vi "logging_start.vi"(8 "error in":errorcluster caption="error in (no error)", 11 "VISA resource name":refnum<visa-resource-name>) -> (0 "error out":errorcluster, 3 "VISA resource name out":refnum<visa-resource-name>)   [LabVIEW 2022 SP3, in "hmp4000_rsidr_core.lvlib"]
uses:
  hmp4000_rsidr_core.lvlib
  _type_Logging_Parameter.ctl
  type_Error_Codes.ctl
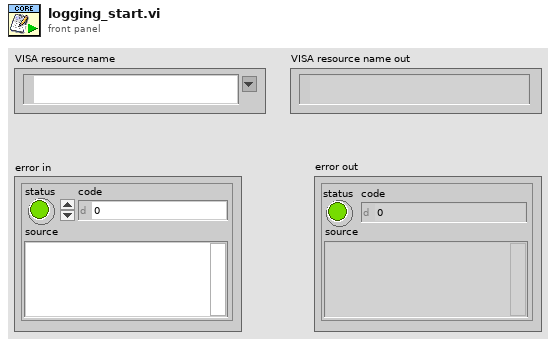
[diagram p1: front panel]
types:
  T1 = typedef "hmp4000_rsidr_core.lvlib/_type_Logging_Parameter.ctl" = enum16{"Type (String)", "SessionAlias(String)", "FormatString (String)", "UDPconectionID (I32)", "UDPlocalPort (I32)", "UDPremotePort (I32)", "UDPremoteHost (String)", "FILEmode (I32)", "FILEpath (String)", "FILEopenID (I32)", "DataMaxLogLen (I32)"}
  T2 = enum16{"open", "replace", "create", "open or create", "replace or create", "replace or create with confirmation"}
  T3 = typedef "hmp4000_rsidr_core.lvlib/type_Error_Codes.ctl" = enum16{"No_error", "VISA_err_ResourceNotFound", "VISA_err_Timeout", "VISA_warn_MoreDataAvailable", "RS_err_MissingCallback", "RS_err_InvalidAttribute", "RS_err_InvalidValue", "RS_err_UnknownResource", "RS_err_AlreadyInitialized", "RS_err_InstrumentStatus", "RS_err_BadRepCapName", "RS_err_TypesMismatch", "RS_err_ValueNotSupported", "RS_err_InvalidRngTable", "RS_err_IDqueryFail", "RS_err_UnexpResponse", "VISA_warn_ConfigNotLoaded", "RS_err_AttributeNotReadable", "RS_err_AttributeNotWritable", "RS_err_InstrumentType", "RS_err_InstrumentOption", "VISA_err_InvalidSize", "RS_err_ReliabilityIndicator", "VISA_warn_UnknownStatus", "VISA_warn_TermCharRead", "VISA_err_IO_error", "RS_err_FunctionNotSupported", "VISA_warn_QueueEmpty"}
  T4 = typedef "hmp4000_rsidr_core.lvlib/type_Session_Data.ctl" = cluster{"IDN string":string, "Instrument FW":string, "Instr type":string, "Instr type for err. msg.":string, "Installed Options":string[], "Ignore Error Messages":string, "Logging params":variant, "OPC Timeout":i32, "VISA Timeout":i32, "STB Poll VISA Timeout":i32, "Additional Flags":i32, "Wait Before Read":i32, "Wait Before Write":i32, "Option String Flags":i32, "IO Segment Size":i64, "VISA Access Mode":T5, "Interface Type":T6, "OPC Wait Mode":T7, "Bin Float Number  Format":T8, "Bin Integer Number Format":T9, "Simulate":bool, "VXIcapable":bool, "Duplicate Session":bool, "Add LF to Write":bool, "Logging":bool, "Fast Sweep":bool, "Query Instrument Status":bool, "Check Range":bool, "Check Options":bool}
  T5 = typedef "hmp4000_rsidr_core.lvlib/type_VisaAccessMode.ctl" = u16
  T6 = typedef "hmp4000_rsidr_core.lvlib/type_InterfaceType.ctl" = enum16{"Unknown", "GPIB", "VXI", "GPIB_VXI", "ASRL", "PXI", "TCPIP", "USB", "SOCKET"}
  T7 = typedef "hmp4000_rsidr_core.lvlib/type_OPC_Wait_Mode.ctl" = enum16{"STBpolling", "STBpollingSlow", "STBpollingSuperSlow", "ServiceRequest", "OPCquery"}
  T8 = typedef "hmp4000_rsidr_core.lvlib/type_Binary_Float_Number_Format.ctl" = enum16{"Float_4_Bytes_Swapped", "Float_4_Bytes", "Double_8_Bytes_Swapped", "Double_8_Bytes"}
  T9 = typedef "hmp4000_rsidr_core.lvlib/type_Binary_Integer_Number_Format.ctl" = enum16{"Int32_4_Bytes_Swapped", "Int32_4 Bytes", "Int16_2_Bytes_Swapped", "Int16_2_Bytes"}
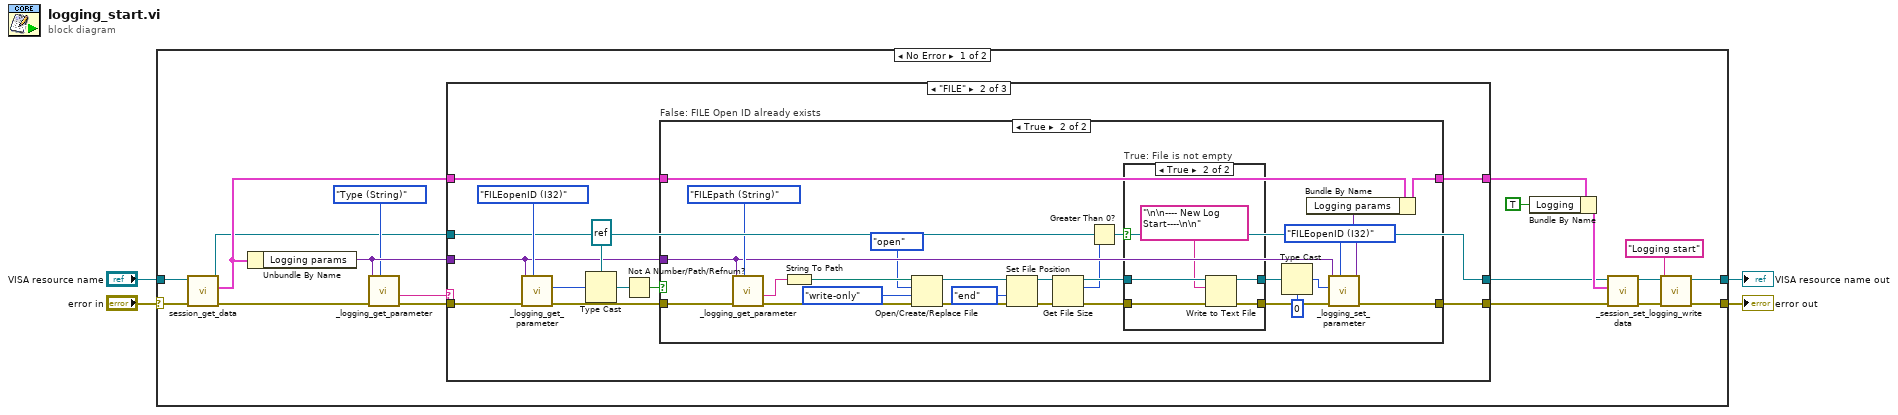
[diagram p0: block diagram]
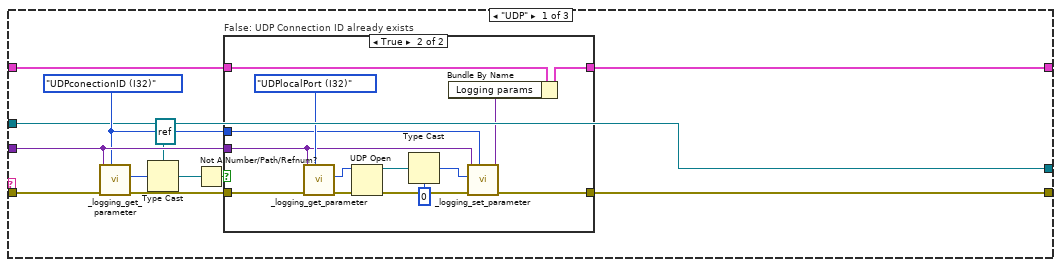
[diagram p2: hidden frame]
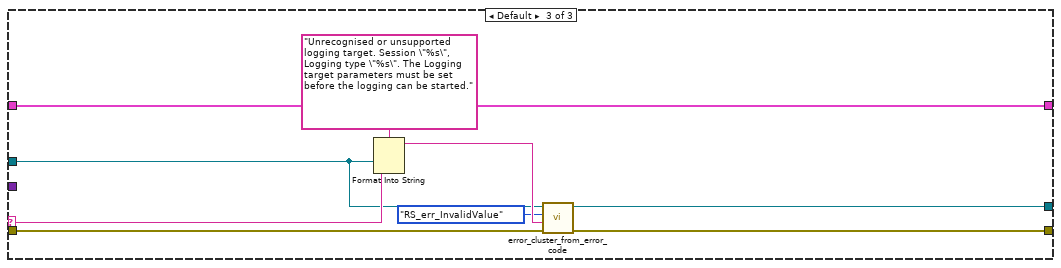
[diagram p6: hidden frame]
diagram:
  n1 = case shown="No Error" "error in" {
    selector: "error in" -> [w23 w109]
    tunnel: [w14 w109] -> w2
    tunnel: "VISA resource name" -> [w22 w108]
    tunnel: [w13 w108] -> w1
    frame No Error {
      n2 = call "session_get_data.vi"("error in"=w23, "VISA resource name"=w22) -> ("error out"=w11:errorcluster, "Session User Data out"=w20:T4, "VISA resource name out"=w5:refnum<visa-resource-name>)  [unwired: 6 in, 1 out]
      n3 = Unbundle By Name(w20) -> ("Logging params"=w10:variant)
      n4 = call "_logging_get_parameter.vi"("Logging Parameter"=_type_Logging_Parameter."Type (String)", "error in"=w11, "Logging params in"=w10) -> ("error out"=w8:errorcluster, "String parameter out"=w7:string)  [unwired: 4 in, 3 out]
      n5 = case shown="\"FILE\"" w7 {
        selector: w7 -> [_ _ w101]
        tunnel: w8 -> [w31 w63 w106]
        tunnel: [w33 w54 w105] -> w21
        tunnel: w20 -> [w34 w57 w104]
        tunnel: [w32 w56 w104] -> w18
        tunnel: w5 -> [w24 w52 w100]
        tunnel: w10 -> [w30 w53 _]
        tunnel: [w24 w52 w102] -> w6
        frame "UDP" {
          w25 = _type_Logging_Parameter."UDPconectionID (I32)" ("Logging Parameter")
          n6 = call "_logging_get_parameter.vi"("Logging Parameter"=w25, "error in"=w31, "Logging params in"=w30) -> ("error out"=w29:errorcluster, "Int32 parameter out"=w28:i32)  [unwired: 4 in, 3 out]
          n7 = Type Cast(type=refnum<k16> refnum ("connection ID"), x=w28) -> (*(type *) &x=w26:refnum<k16>)
          n8 = Not A Number/Path/Refnum?(number/path/refnum=w26) -> (NaN/Path/Refnum?=w35:bool)
          n9 = case "False: UDP Connection ID already exists" shown="True" w35 {
            tunnel: w29 -> [w37 w51]
            tunnel: [w37 w46] -> w33
            tunnel: w34 -> [w36 w40]
            tunnel: [w36 w39] -> w32
            tunnel: w30 -> [_ w45]
            tunnel: w25 -> [_ w43]
            frame False {
            }
            frame True {
              n10 = call "_logging_get_parameter.vi"("Logging Parameter"=_type_Logging_Parameter."UDPlocalPort (I32)", "error in"=w51, "Logging params in"=w45) -> ("error out"=w50:errorcluster, "Int32 parameter out"=w48:i32)  [unwired: 4 in, 3 out]
              n11 = UDP Open(8:w50, 11:w48) -> (port=w38:refnum<k16>, 0:w47:errorcluster)  [unwired: 1 in, 3 out]
              n12 = Type Cast(type=0, x=w38) -> (*(type *) &x=w41:i32)
              n13 = call "_logging_set_parameter.vi"("Logging Parameter"=w43, "error in"=w47, "Int32 parameter (0)"=w41, "Logging params in"=w45) -> ("error out"=w46:errorcluster, "Logging params out"=w44:variant)  [unwired: 6 in]
              n14 = Bundle By Name(cluster=w40, "Logging params"=w44) -> (w39:T4)
            }
          }
        }
        frame "FILE" {
          n15 = call "_logging_get_parameter.vi"("Logging Parameter"=_type_Logging_Parameter."FILEopenID (I32)", "error in"=w63, "Logging params in"=w53) -> ("error out"=w59:errorcluster, "Int32 parameter out"=w60:i32)  [unwired: 4 in, 3 out]
          n16 = Type Cast(type=refnum<file> refnum ("refnum out"), x=w60) -> (*(type *) &x=w62:refnum<file>)
          n17 = Not A Number/Path/Refnum?(number/path/refnum=w62) -> (NaN/Path/Refnum?=w58:bool)
          n18 = case "False: FILE Open ID already exists" shown="True" w58 {
            tunnel: w59 -> [w65 w88]
            tunnel: w57 -> [w64 w91]
            tunnel: [w64 w90] -> w56
            tunnel: [w65 w80] -> w54
            tunnel: w53 -> [_ w85]
            frame False {
            }
            frame True {
              n19 = call "_logging_get_parameter.vi"("Logging Parameter"=_type_Logging_Parameter."FILEpath (String)", "error in"=w88, "Logging params in"=w85) -> ("error out"=w75:errorcluster, "String parameter out"=w66:string)  [unwired: 4 in, 3 out]
              n20 = String To Path(string=w66) -> (path=w86:path)
              n21 = Open/Create/Replace File(file path (use dialog)=w86, error in=w75, operation (0:open)=T2."open", access (0:read/write)=enum16{"read/write", "read-only", "write-only"}."write-only") -> (refnum out=w78:refnum<file>, error out=w77:errorcluster)  [unwired: 2 in, 1 out]
              n22 = Set File Position(refnum=w78, from (0:start)=enum16{"start", "end", "current"}."end", error in=w77) -> (refnum out=w71:refnum<file>, error out=w72:errorcluster)  [unwired: 1 in]
              n23 = Get File Size(file=w71, error in=w72) -> (refnum out=w70:refnum<file>, size (in bytes)=w67:i64, 0:w69:errorcluster)
              n24 = Greater Than 0?(x=w67) -> (x > 0?=w68:bool)
              n25 = case "True: File is not empty" shown="True" w68 {
                tunnel: w69 -> [w92 w98]
                tunnel: w70 -> [w93 w97]
                tunnel: [w92 w96] -> w74
                tunnel: [w93 w95] -> w73
                frame False {
                }
                frame True {
                  n26 = Write to Text File(file (use dialog)=w97, text="\n\n---- New Log Start----\n\n", error in=w98) -> (refnum out=w95:refnum<file>, error out=w96:errorcluster)  [unwired: 1 in, 1 out]
                }
              }
              n27 = Type Cast(type=0, x=w73) -> (*(type *) &x=w81:i32)
              n28 = call "_logging_set_parameter.vi"("Logging Parameter"=_type_Logging_Parameter."FILEopenID (I32)", "error in"=w74, "Int32 parameter (0)"=w81, "Logging params in"=w85) -> ("error out"=w80:errorcluster, "Logging params out"=w84:variant)  [unwired: 6 in]
              n29 = Bundle By Name(cluster=w91, "Logging params"=w84) -> (w90:T4)
            }
          }
        }
        frame Default {
          n30 = Format Into String(format string="Unrecognised or unsupported logging target. Session \"%s\", Logging type \"%s\". The Logging target parameters must be set before the logging can be started.", w100, w101) -> (resulting string=w103:string)  [unwired: 2 in, 1 out]
          n31 = call "error_cluster_from_error_code.vi"("error in"=w106, "Error Message (\"\")"=w103, "Error Enum in"=type_Error_Codes."RS_err_InvalidValue", "VISA resource name"=w100) -> ("error out"=w105:errorcluster, "VISA resource name out"=w102:refnum<visa-resource-name>)  [unwired: 6 in]
        }
      }
      n32 = Bundle By Name(cluster=w18, "Logging"=TRUE) -> (w17:T4)
      n33 = call "_session_set_data.vi"("error in"=w21, "Session User Data in"=w17, "VISA resource name"=w6) -> ("error out"=w16:errorcluster, "VISA resource name out"=w15:refnum<visa-resource-name>)  [unwired: 7 in]
      n34 = call "logging_write.vi"("error in"=w16, "String to write"="Logging start", "VISA resource name"=w15) -> ("error out"=w14:errorcluster, "VISA resource name out"=w13:refnum<visa-resource-name>)  [unwired: 7 in]
    }
    frame Error {
    }
  }
  "VISA resource name out" <- w1
  "error out" <- w2
